vi "FloatToHex.vi"(11 "浮点数":sgl[](array[numeric])) -> (3 "DCBA整形输出":u16[](array[numeric]) format="%04xH")   [LabVIEW 2016, in "挥发酚.lvlib"]
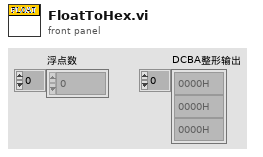
[diagram p1: front panel]
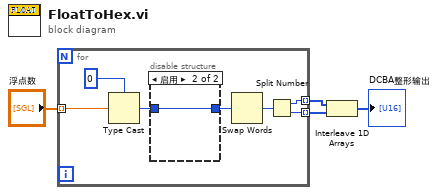
[diagram p0: block diagram]
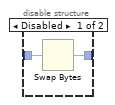
[diagram p2: hidden frame]
diagram:
  n1 = for {
    tunnel: "浮点数" -> [w9] mode=indexing
    tunnel: [w8] -> w2 mode=indexing
    tunnel: [w7] -> w3 mode=indexing
    n2 = Type Cast(type=0, x=w9) -> (*(type *) &x=w6:i32)
    n3 = disable-structure shown="启用" {
      disable-tunnel: w6 -> [w13 w14]
      disable-tunnel: [w12 w14] -> w5
      frame Disabled {
        n4 = Swap Bytes(anything=w13) -> (byte swapped=w12:i32)
      }
      frame Enabled {
      }
    }
    n5 = Swap Words(1:w5) -> (0:w11:i32)
    n6 = Split Number(x=w11) -> (hi(x)=w8:u16, lo(x)=w7:u16)
  }
  n7 = Interleave 1D Arrays(w2, w3) -> (→"DCBA整形输出":u16[])
